vi "constants_HL.vi"(4 "whichMotors 3":i32[](array[numeric]), 6 "nMotors 3":i32, 7 "whichMotors 2":i32[](array[numeric]), 8 "nMotors 2":i32, 9 "whichMotors 1":i32[](array[numeric]), 10 "nMotors 1":i32, 11 "nMotors":i32) -> (3 "Constants HL":T1={"Frame Points"=[], "Brace Points in P"=[], "QP_lb"=[], "QP_ub"=[], "Q for QP"=[], "nMotors"=0, "QP stopping criteria"={"function tolerance"=1e-08, "parameter tolerance"=1000000.0, "max iterations"=10000, "max function calls"=10000, "gradient tolerance"=1000000.0, "max time (sec)"=-1.0}, "MotorsPos_wrt_Markers"=[], "nMotors 1"=0, "nMotors 2"=0, "MotorsPos_wrt_Markers pel"=[], "Frame Points_pel"=[], "Brace Points in P_pel"=[], "QP_lb pel"=[], "QP_ub pel"=[], "Q for QP pel"=[], "MotorsPos_wrt_Markers knees"=[], "nMotors 3"=0})   [LabVIEW 2017]
uses:
  typeDef/constants_HL.ctl
  <vilib>/gmath/NumericalOptimization/stopping criteria.ctl
  <vilib>/Analysis/7linalg.llb/Create Special Real Matrix.vi
  <vilib>/Analysis/Matrix/Numeric/Conversions/Matrix To Array - RM.vi
  <vilib>/Analysis/NI_AALPro.lvlib
  <vilib>/Analysis/Matrix/NI_Matrix.lvlib
  <vilib>/gmath/NI_Gmath.lvlib
panel:
  in  "QP stopping criteria":T2={"function tolerance"=1e-08, "parameter tolerance"=1000000.0, "max iterations"=10000, "max function calls"=10000, "gradient tolerance"=1000000.0, "max time (sec)"=-1.0}
  in  "Constants HL":T1={"Frame Points"=[], "Brace Points in P"=[], "QP_lb"=[], "QP_ub"=[], "Q for QP"=[], "nMotors"=0, "QP stopping criteria"={"function tolerance"=1e-08, "parameter tolerance"=1000000.0, "max iterations"=10000, "max function calls"=10000, "gradient tolerance"=1000000.0, "max time (sec)"=-1.0}, "MotorsPos_wrt_Markers"=[], "nMotors 1"=0, "nMotors 2"=0, "MotorsPos_wrt_Markers pel"=[], "Frame Points_pel"=[], "Brace Points in P_pel"=[], "QP_lb pel"=[], "QP_ub pel"=[], "Q for QP pel"=[], "MotorsPos_wrt_Markers knees"=[], "nMotors 3"=0}
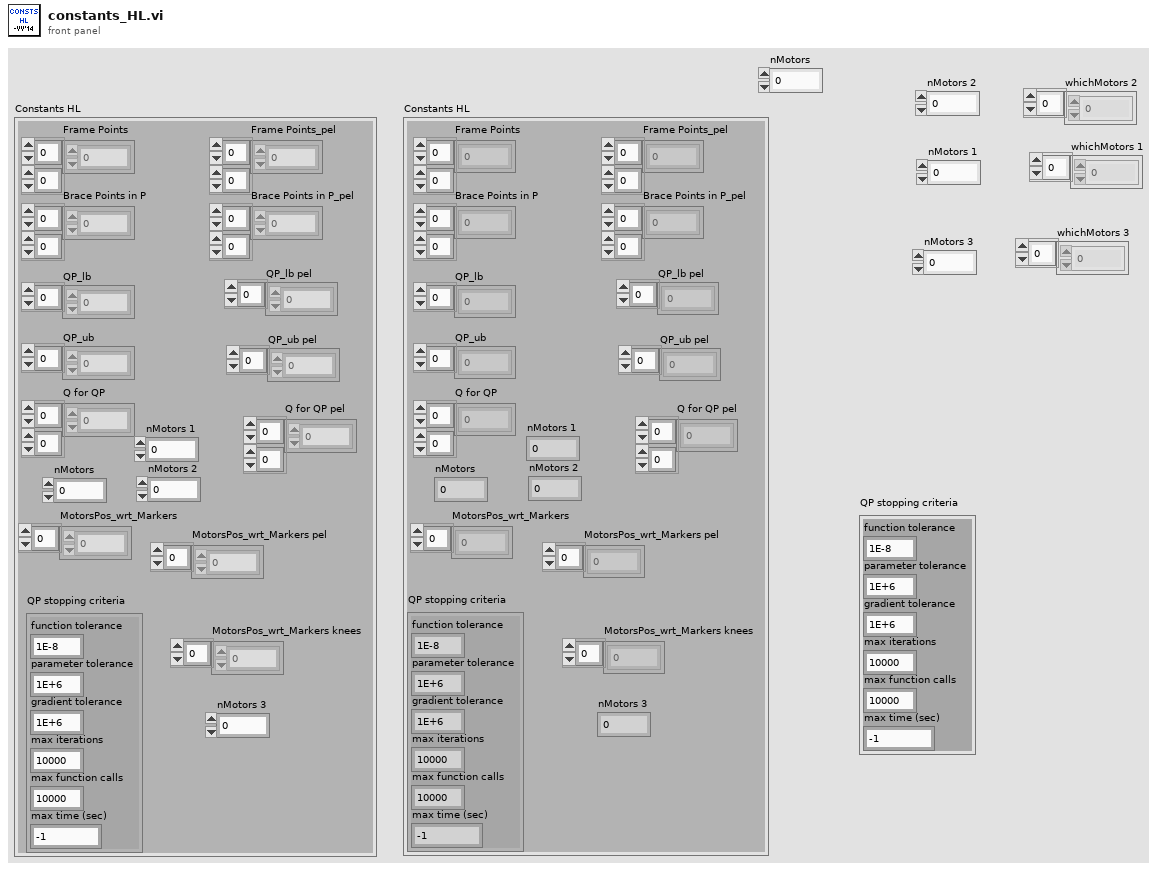
[diagram p1: front panel]
types:
  T1 = typedef "constants_HL.ctl" = cluster{"Frame Points":dbl[][], "Brace Points in P":dbl[][], "QP_lb":dbl[], "QP_ub":dbl[], "Q for QP":dbl[][], "nMotors":i32, "QP stopping criteria":T2, "MotorsPos_wrt_Markers":i32[], "nMotors 1":i32, "nMotors 2":i32, "MotorsPos_wrt_Markers pel":i32[], "Frame Points_pel":dbl[][], "Brace Points in P_pel":dbl[][], "QP_lb pel":dbl[], "QP_ub pel":dbl[], "Q for QP pel":dbl[][], "MotorsPos_wrt_Markers knees":i32[], "nMotors 3":i32}
  T2 = typedef "NI_Gmath.lvlib/stopping criteria.ctl" = cluster{"function tolerance":dbl, "parameter tolerance":dbl, "max iterations":i32, "max function calls":i32, "gradient tolerance":dbl, "max time (sec)":dbl}
  T3 = typedef "NI_Matrix.lvlib/RealMatrix.ctl" = dbl[][]
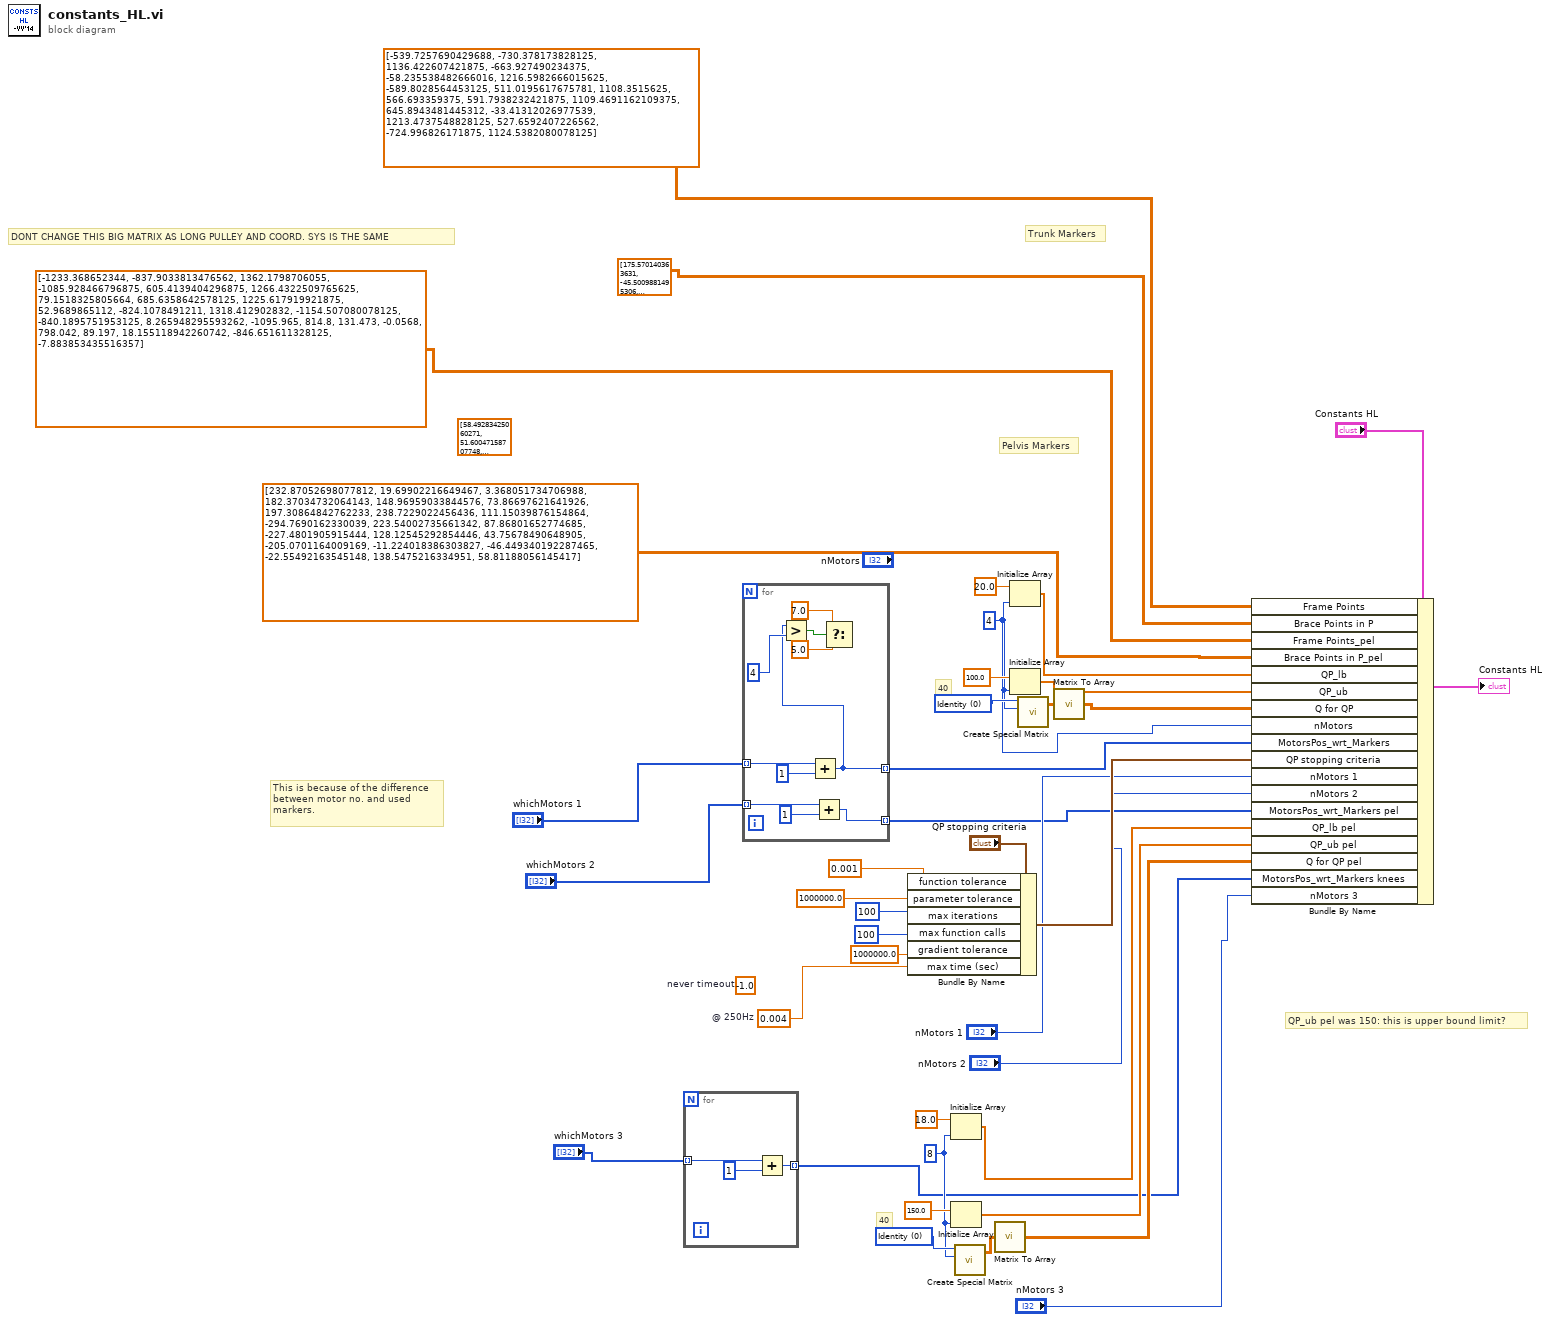
[diagram p0: block diagram]
diagram:
  (unwired) dbl[][] [[58.49283425060271, 51.60047158707748, -12.536354960473588], [166.4800786367168, 122.38817262319624, 37.430060403830666], [163.76961896274278, 206.46120052126622, 52.76503430024542], [-112.4912149072848, 249.303580216435, 53.337782928542424], [-136.06093587909956, 146.95936163023086, 28.727554555221637], [-56.06842114267545, 50.31278861299169, -17.64631317985034], [15.209571378808638, 134.67376712671356, 33.078807479526155]] ("MarksInP 2")
  w9 = 8 ("dimension size")
  w13 = 0 items=["Identity", "Diagonal", "Toepliz", "Vandermonde", "Companion", "Hankel", "Hadamard", "Wilkinson", "Hilbert", "Inverse Hilbert", "Rosser", "Pascal"] ("matrix type")
  w15 = 4 ("dimension size")
  w17 = 0.004  # @ 250Hz
  w31 = 0 items=["Identity", "Diagonal", "Toepliz", "Vandermonde", "Companion", "Hankel", "Hadamard", "Wilkinson", "Hilbert", "Inverse Hilbert", "Rosser", "Pascal"] ("matrix type")
  (unwired) -1.0  # never timeout
  # "QP_ub pel was 150: this is upper bound limit?"
  # "DONT CHANGE THIS BIG MATRIX AS LONG PULLEY AND COORD. SYS IS THE SAME"
  # "40"
  # "Pelvis Markers"
  # "Trunk Markers"
  # "40"
  # "This is because of the difference\nbetween motor no. and used\nmarkers."
  n1 = for {
    tunnel: "whichMotors 3" -> [w41] mode=indexing
    tunnel: [w40] -> w3 mode=indexing
    n2 = Add(x=w41, y=1) -> (x+y=w40:i32)
  }
  n3 = for {
    tunnel: "whichMotors 1" -> [w50] mode=indexing
    tunnel: [w46] -> w25 mode=indexing
    tunnel: "whichMotors 2" -> [w44] mode=indexing
    tunnel: [w43] -> w20 mode=indexing
    n4 = Add(x=w50, y=1) -> (x+y=w46:i32)
    n5 = Greater?(x=w46, y=4 ("x")) -> (0:w49:bool)
    n6 = Add(x=w44, y=1) -> (x+y=w43:i32)
    n7 = Select(t=7.0, s=w49, f=5.0) -> ()  [unwired: 1 out]
  }
  n8 = Bundle By Name(cluster="QP stopping criteria", "function tolerance"=0.001, "parameter tolerance"=1000000.0, "max iterations"=100, "max function calls"=100, "gradient tolerance"=1000000.0, "max time (sec)"=w17) -> (w27:T2)
  n9 = Initialize Array(18.0 ("t"), w9) -> (w8:dbl[])
  n10 = Initialize Array(150.0 ("element"), w9) -> (w7:dbl[])
  n11 = call-poly <vilib>:"Create Special Matrix.vi"("matrix type"=w13, "matrix size"=w9) -> ("Special Matrix"=w12:T3)  [unwired: 3 in, 1 out]
  n12 = call-poly <vilib>:"Matrix To Array.vi"("Real Matrix"=w12) -> ("Real 2D Array"=w6:dbl[][])
  n13 = Initialize Array(20.0 ("t"), w15) -> (w14:dbl[])
  n14 = Initialize Array(100.0 ("element"), w15) -> (w32:dbl[])
  n15 = call-poly <vilib>:"Create Special Matrix.vi"("matrix type"=w31, "matrix size"=w15) -> ("Special Matrix"=w30:T3)  [unwired: 3 in, 1 out]
  n16 = call-poly <vilib>:"Matrix To Array.vi"("Real Matrix"=w30) -> ("Real 2D Array"=w29:dbl[][])
  n17 = Bundle By Name(cluster="Constants HL", "Frame Points"=dbl[][] [[-539.7257690429688, -730.378173828125, 1136.422607421875], [-663.927490234375, -58.235538482666016, 1216.5982666015625], [-589.8028564453125, 511.0195617675781, 1108.3515625], [566.693359375, 591.7938232421875, 1109.4691162109375], [645.8943481445312, -33.41312026977539, 1213.4737548828125], [527.6592407226562, -724.996826171875, 1124.5382080078125]] ("Frame Coords"), "Brace Points in P"=dbl[][] [[175.570140363631, -45.5009881495306, -30.46789487634584], [163.45363570663963, 116.77586032564005, 69.63751596179411], [198.1614608420813, 270.60775566408194, 106.34548116514465], [-169.11904144769582, 313.9760777177392, 96.08600909789396], [-160.29331326326255, 150.49068766079037, 42.505103690046255], [-177.4253347080142, -13.664735487376138, -40.746881456420574], [1.5801612216885514, 133.6332739932152, 56.07130982592019]] ("MarksInP"), "Frame Points_pel"=dbl[][] [[-1233.368652344, -837.9033813476562, 1362.1798706055], [-1085.928466796875, 605.4139404296875, 1266.4322509765625], [79.1518325805664, 685.6358642578125, 1225.617919921875], [52.9689865112, -824.1078491211, 1318.412902832], [-1154.507080078125, -840.1895751953125, 8.265948295593262], [-1095.965, 814.8, 131.473], [-0.0568, 798.042, 89.197], [18.155118942260742, -846.651611328125, -7.883853435516357]] ("Frame Coords 2"), "Brace Points in P_pel"=dbl[][] [[232.87052698077812, 19.69902216649467, 3.368051734706988], [182.37034732064143, 148.96959033844576, 73.86697621641926], [197.30864842762233, 238.7229022456436, 111.15039876154864], [-294.7690162330039, 223.54002735661342, 87.86801652774685], [-227.4801905915444, 128.12545292854446, 43.75678490648905], [-205.0701164009169, -11.224018386303827, -46.449340192287465], [-22.55492163545148, 138.5475216334951, 58.81188056145417]] ("MarksInP 2"), "QP_lb"=w14, "QP_ub"=w32, "Q for QP"=w29, "nMotors"=w15, "MotorsPos_wrt_Markers"=w25, "QP stopping criteria"=w27, "nMotors 1"="nMotors 1", "nMotors 2"="nMotors 2", "MotorsPos_wrt_Markers pel"=w20, "QP_lb pel"=w8, "QP_ub pel"=w7, "Q for QP pel"=w6, "MotorsPos_wrt_Markers knees"=w3, "nMotors 3"="nMotors 3") -> (→"Constants HL":T1)
